vi "Is Voltage Datas Out Range.vi"(8 "error in (no error)":errorcluster, 11 "channel":i8) -> (0 "error out":errorcluster, 3 "function return":i32)   [LabVIEW 2021, in "vmmso.lvlib"]
doc: "DLL_API int WINAPI IsVoltageDatasOutRange(char channel);"
uses:
  vmmso.lvlib
  vmmso.dll
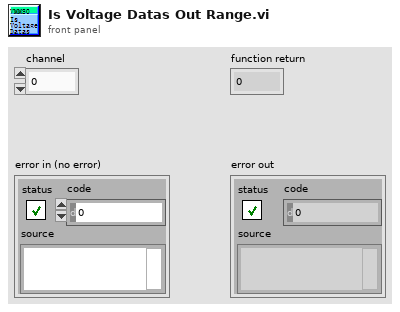
[diagram p1: front panel]
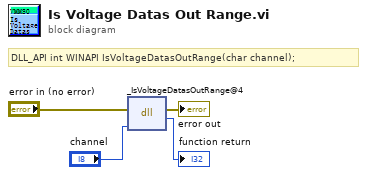
[diagram p0: block diagram]
diagram:
  # "DLL_API int WINAPI IsVoltageDatasOutRange(char channel);"
  n1 = dll-call lib="O:/MSO/library/demo-Labview/vmmso/vmmso.*" fn="_IsVoltageDatasOutRange@4"(error in="error in (no error)", "channel"="channel") -> (error out=→"error out":errorcluster, →"function return":i32)  [unwired: 3 in, 1 out]
